vi "Get Messaging Client List.vi"(8 "error in (no error)":errorcluster, 11 "VolatusAPI in":refnum<class "VolatusAPI.lvclass">) -> (0 "error out":errorcluster, 2 "Client List":T1, 3 "VolatusAPI out":refnum<class "VolatusAPI.lvclass">)   [LabVIEW 2020, in "Volatus.lvlib" / "VolatusAPI.lvclass"]
uses:
  VolatusAPI.lvclass
  messages/TcpClientList/Data.ctl
  messages/TcpClientInfo/Data.ctl
  VolatusAPI.lvclass/VolatusAPI.ctl
  lv-vecto/Vecto/TCPMessageService/TCPMessageAPI.lvclass/TCPMessageAPI.ctl
  lv-vecto/Vecto/TCPMessageService/TCPMessageAPI.lvclass
  messages/TcpClientInfo/TcpClientInfo.lvlib
  messages/TcpClientList/TcpClientList.lvlib
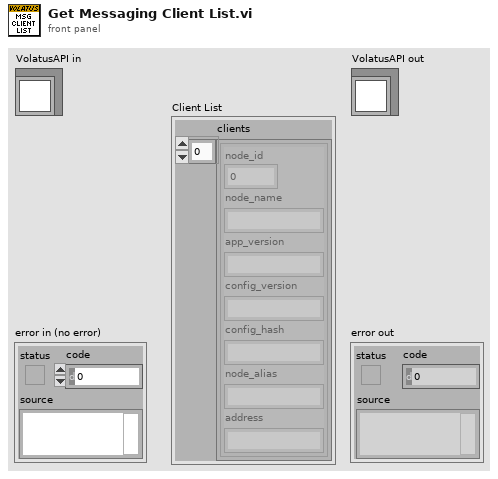
[diagram p1: front panel]
types:
  T1 = typedef "TcpClientList.lvlib/Data.ctl" = cluster{"clients":T2[]}
  T2 = typedef "TcpClientInfo.lvlib/Data.ctl" = cluster{"node_id":u32, "node_name":string, "app_version":string, "config_version":string, "config_hash":string, "node_alias":string, "address":string}
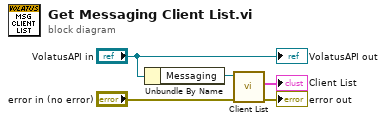
[diagram p0: block diagram]
diagram:
  n1 = Unbundle By Name("VolatusAPI in") -> ("Messaging"=w4:refnum<class "TCPMessageAPI.lvclass">)
  n2 = call "Client List.vi"("error in (no error)"="error in (no error)", "TCPMessageAPI in"=w4) -> ("error out"=→"error out":errorcluster, "Client List"=→"Client List":T1)  [unwired: 7 in, 1 out]
  "VolatusAPI out" <- "VolatusAPI in"
